vi "GA Set Trap Prm.vi"(8 "error in (no error)":errorcluster caption="错误输入（无错误）", 10 "pPrm":T1, 11 "nAxisNum":i16) -> (0 "error out":errorcluster caption="错误输出", 2 "pPrm out":T1, 3 "function return":i32)   [LabVIEW 2024, in "GAS.lvlib"]
doc: "extern \"C\" __declspec(dllimport) int GA_SetTrapPrm(short nAxisNum,TTrapPrm *pPrm);"
uses:
  GAS.lvlib
  GAS.dll
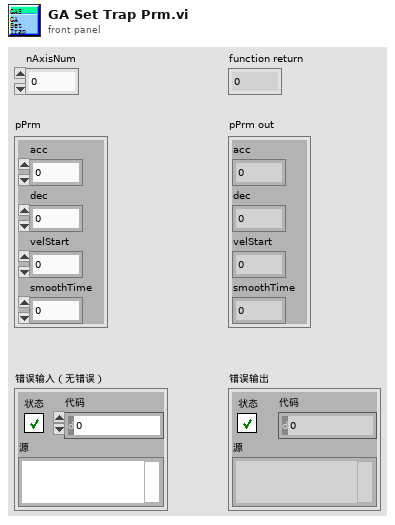
[diagram p1: front panel]
types:
  T1 = cluster{"acc":dbl, "dec":dbl, "velStart":dbl, "smoothTime":i16}
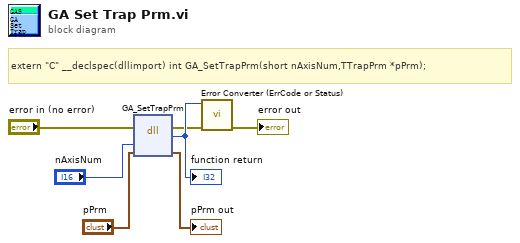
[diagram p0: block diagram]
diagram:
  # "extern \"C\" __declspec(dllimport) int GA_SetTrapPrm(short nAxisNum,TTrapPrm *pPrm);"
  n1 = dll-call lib="PTH2?abs D实验室软件（勿删）集成测试系统GAS.*" fn="GA_SetTrapPrm"(error in="error in (no error)", "nAxisNum"="nAxisNum", "pPrm"="pPrm") -> (error out=w2:errorcluster, w7:i32, "pPrm"=→"pPrm out":T1)  [unwired: 3 in, 1 out]
  "function return" <- w7
  n2 = call "Error Converter (ErrCode or Status).vi"("error in (no error)"=w2, "error code"=w7) -> ("error out"=→"error out":errorcluster)  [unwired: 9 in]
